vi "ATF Storage-Get Recoverable Network Streams Errors_R.vi"() -> (3 "recoverable network streams errors":i32[](array[numeric]))   [LabVIEW 2022 SP3]
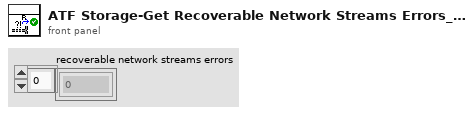
[diagram p1: front panel]
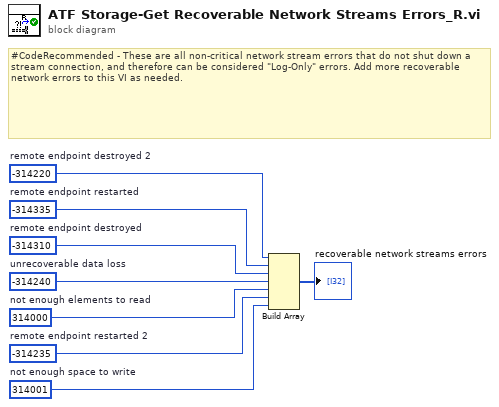
[diagram p0: block diagram]
diagram:
  w8 = -314220  # remote endpoint destroyed 2
  w6 = 314001  # not enough space to write
  w4 = 314000  # not enough elements to read
  w5 = -314235  # remote endpoint restarted 2
  w3 = -314240  # unrecoverable data loss
  w2 = -314310  # remote endpoint destroyed
  w1 = -314335  # remote endpoint restarted
  # "#CodeRecommended - These are all non-critical network stream errors that do not shut down a stream connection, and therefore can be considered \"Log-Only\" errors. Add more recoverable network errors to this VI as needed."
  n1 = Build Array(w8, w1, w2, w3, w4, w5, w6) -> (→"recoverable network streams errors":i32[])
